vi "sendRequest.vi"(7 "TaskName":string, 8 "error in (no error)":errorcluster, 9 "Parameters":variant, 10 "Request":string, 11 "pdbm_testsys_reqst_event":refnum<user-event>) -> (0 "error IO":errorcluster, 3 "pdbm_testsys_reqst_event out":refnum<user-event>)   [LabVIEW 2015, in "pdbm_test_system.lvlib"]
uses:
  pdbm_test_system.lvlib
  pdbm_testsys_taskroute_inter/UsrDefine/pdbm_testsys_reqst_data.ctl
  pdbm_testsys_taskroute_inter/pdbm_testsys_taskroute_inter.lvlib
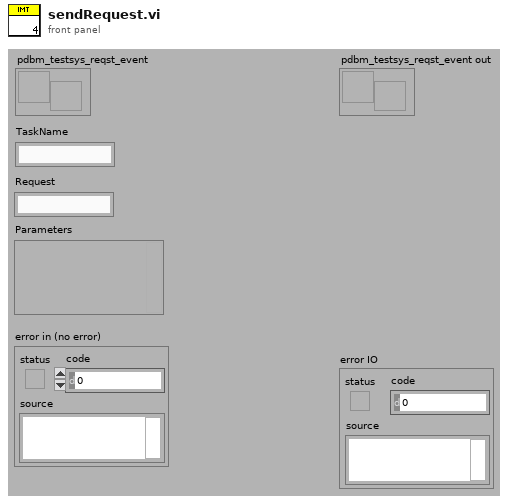
[diagram p1: front panel]
types:
  T1 = cluster{"TaskName":string, "Request":string, "Parameters":variant}
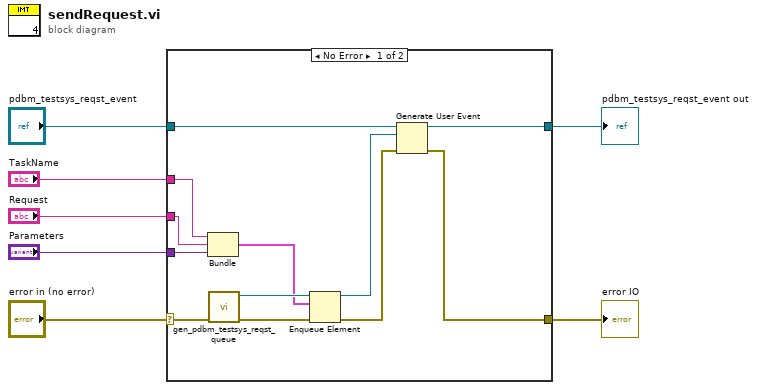
[diagram p0: block diagram]
diagram:
  n1 = case shown="No Error" "error in (no error)" {
    selector: "error in (no error)" -> [w19 w21]
    tunnel: "pdbm_testsys_reqst_event" -> [w16 w20]
    tunnel: [w13 w20] -> w5
    tunnel: [w8 w21] -> w4
    tunnel: "TaskName" -> [w10 _]
    tunnel: "Request" -> [w11 _]
    tunnel: "Parameters" -> [w12 _]
    frame No Error {
      n2 = Bundle("TaskName"=w10, "Request"=w11, "Parameters"=w12) -> (w9:T1)  [unwired: 1 in]
      n3 = call "gen_pdbm_testsys_reqst_queue.vi"("error in (no error)"=w19) -> ("error IO"=w18:errorcluster, "pdbm_testsys_reqst_event"=w17:refnum<queue>)  [unwired: 9 in]
      n4 = Enqueue Element(queue=w17, element=w9, error in (no error)=w18) -> (queue out=w14:refnum<queue>, error out=w15:errorcluster)  [unwired: 1 in, 1 out]
      n5 = Generate User Event(user event=w16, event data cluster=w14, error in=w15) -> (user event out=w13:refnum<user-event>, error out=w8:errorcluster)  [unwired: 1 in]
    }
    frame Error {
    }
  }
  "pdbm_testsys_reqst_event out" <- w5
  "error IO" <- w4
